vi "Read Alarm Output.vi"(0 "VISA resource name":refnum<visa-resource-name>, 1 "Unit Address (1)":u8=1 min=1 max=254, 5 "Alarm Number (1)":u16=1 min=1 max=4, 11 "error in (no error)":errorcluster) -> (4 "VISA resource name out":refnum<visa-resource-name>, 6 "Alarm Output":bool, 15 "error out":errorcluster)   [LabVIEW 2010, in "Eurotherm 32xx Series.lvlib"]
doc: "This VI reads Alarm output value."
uses:
  <instrlib>/Eurotherm 32xx Series/Eurotherm 32xx Series.lvlib
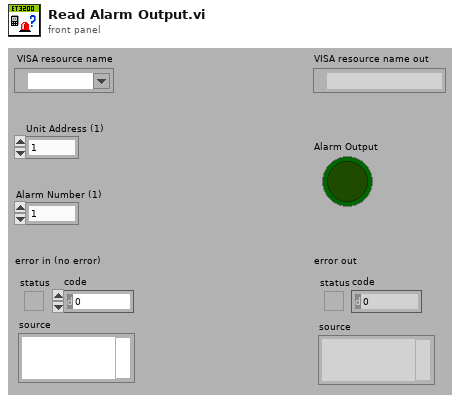
[diagram p1: front panel]
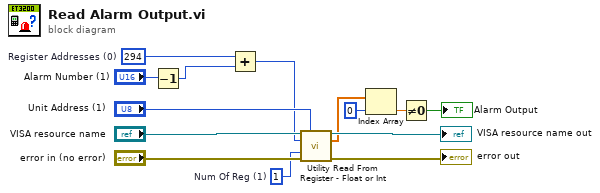
[diagram p0: block diagram]
diagram:
  w9 = u16 1  # Num Of Reg (1)
  w3 = 294  # Register Addresses (0)
  n1 = Decrement(x="Alarm Number (1)") -> (x-1=w2:u16)
  n2 = Add(x=w3, y=w2) -> (x+y=w1:i32)
  n3 = call <instrlib>:"Utility Read From Register - Float or Int.vi"("VISA resource name"="VISA resource name", "Unit Address (1)"="Unit Address (1)", "Register Address (0)"=w1, "Num Of Reg (1)"=w9, "error in (no error)"="error in (no error)") -> ("VISA resource name out"=→"VISA resource name out":refnum<visa-resource-name>, "Data"=w8:sgl[], "error out"=→"error out":errorcluster)  [unwired: 8 in]
  n4 = Index Array(array=w8, index=0) -> (element=w6:sgl)
  n5 = Not Equal To 0?(x=w6) -> (x != 0?=→"Alarm Output":bool)
